vi "configure.vi"(8 "error in (no error)":errorcluster, 10 "Protocol Parameters":T1={"VISA resource name"="", "Baud Rate"=9600, "Data Bits"=8, "Parity"=enum."None", "Flow Control"=0, "Stop Bits"=10, "Timeout (ms)"=10000} {"Stop Bits" items=["1.0"=10, "1.5"=15, "2.0"=20]; "Flow Control" items=["None", "XON/XOFF", "RTS/CTS", "XON/XOFF & RTS/CTS", "DTR/DSR", "XON/XOFF & DTR/DSR"]; "Data Bits" min=5 max=8 step=1}, 11 "SerialProtocol in":refnum<class "SerialProtocol.lvclass">) -> (0 "error out":errorcluster, 3 "SerialProtocol out":refnum<class "SerialProtocol.lvclass">)   [LabVIEW 2013, in "SerialProtocols.lvlib" / "SerialProtocol.lvclass"]
uses:
  <userlib>/Common/SerialProtocols/SerialProtocol/SerialProtocol/SerialProtocol.lvclass
  <userlib>/Common/SerialProtocols/Configuration/ProtocolParameters.ctl
  <userlib>/Common/SerialProtocols/SerialProtocols.lvlib
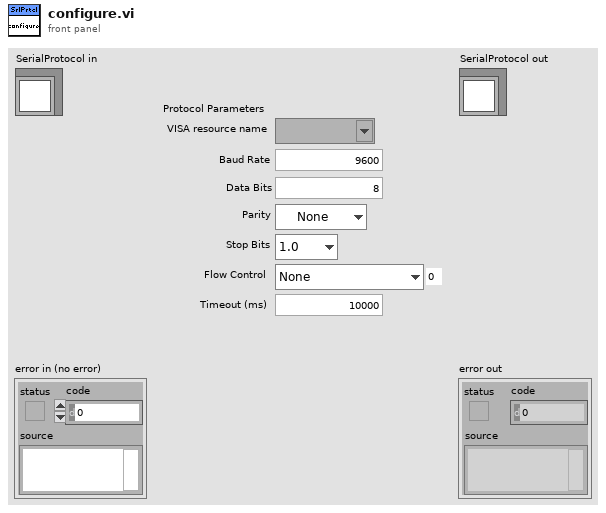
[diagram p1: front panel]
types:
  T1 = typedef "SerialProtocols.lvlib/ProtocolParameters.ctl" = cluster{"VISA resource name":refnum<visa-resource-name>, "Baud Rate":u32, "Data Bits":u16, "Parity":enum16{"None", "Odd", "Even", "Mark", "Space"}, "Flow Control":u16, "Stop Bits":u16, "Timeout (ms)":u32}
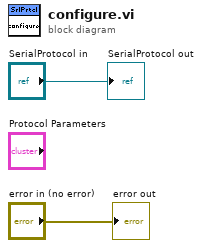
[diagram p0: block diagram]
diagram:
  "error out" <- "error in (no error)"
  "SerialProtocol out" <- "SerialProtocol in"
